vi "Write Comp Driver State.vi"(8 "error in (no error)":errorcluster, 10 "Comp Driver State":T1, 11 "Comp Driver in":refnum<class "Comp Driver.lvclass">) -> (0 "error out":errorcluster, 3 "Comp Driver out":refnum<class "Comp Driver.lvclass">)   [LabVIEW 2014, in "Comp Driver.lvlib" / "Comp Driver.lvclass"]
uses:
  Comp Driver.lvclass
  Comp Driver State.ctl
  <vilib>/Rock Robotics/WPI/Joystick/WPI_JoystickDevRef.ctl
  <vilib>/Rock Robotics/WPI/Joystick/WPI_JoystickDeviceEnum.ctl
  Comp Driver.lvclass/Comp Driver.ctl
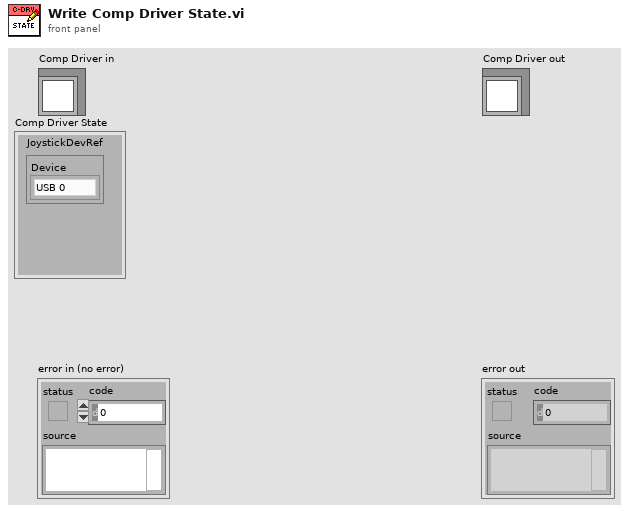
[diagram p1: front panel]
types:
  T1 = typedef "Comp Driver.lvlib/Comp Driver.lvclass/Comp Driver State.ctl" = cluster{"JoystickDevRef":T2}
  T2 = typedef "WPI_JoystickDevRef.ctl" = cluster{"Device":T3}
  T3 = typedef "WPI_JoystickDeviceEnum.ctl" = enum16{"USB 0", "USB 1", "USB 2", "USB 3", "USB 4", "USB 5"}
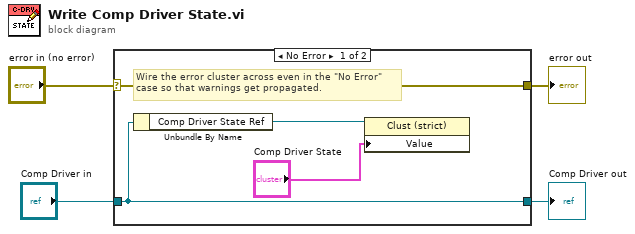
[diagram p0: block diagram]
diagram:
  n1 = case shown="No Error" "error in (no error)" {
    selector: "error in (no error)" -> [w8 w10]
    tunnel: [w8 w10] -> w3
    tunnel: [w7 w9] -> w1
    tunnel: "Comp Driver in" -> [w7 w9]
    frame No Error {
      # "Wire the error cluster across even in the \"No Error\"\ncase so that warnings get propagated."
      n2 = Unbundle By Name(w7) -> ("Comp Driver State Ref"=w6:refnum<vi>)
      n3 = property class="Clust (strict)"(reference=w6, "Value"="Comp Driver State") -> ()  [unwired: 1 in, 2 out]
    }
    frame Error {
    }
  }
  "error out" <- w3
  "Comp Driver out" <- w1
